vi "Get Loaded Instrument Configurations.vi"(8 "Error In":errorcluster) -> (0 "Error Out":errorcluster, 1 "Instrument Configurations":refnum<class "Config from JSON.lvclass">[](array[class]), 2 "Identifiers":string[](array[string]))   [LabVIEW 2020, in "Instrument Manager.lvclass"]
uses:
  Instrument Manager.lvclass
  Instrument Manager.lvclass/Instrument Manager.ctl
  Config from JSON/Config from JSON.lvclass
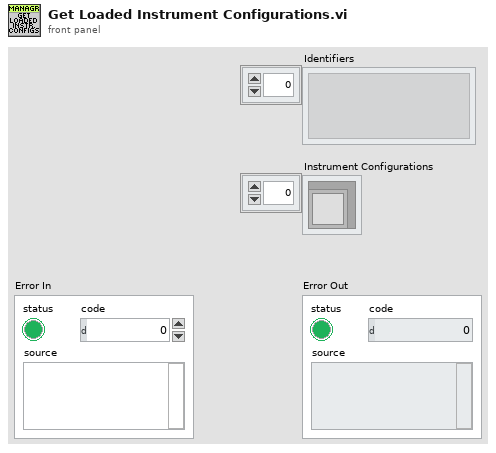
[diagram p1: front panel]
types:
  T1 = typedef "Instrument Manager.lvclass/ObjectAttributes.ctl" = cluster{"ICreate Action Point":refnum<class "ICreate Action Point.lvclass">, "IInstruments":map{string, refnum<class "IInstrument.lvclass">}, "IVirtual Instruments":map{string, refnum<class "IVirtual Instrument.lvclass">}, "Instrument Configurations":map{string, refnum<class "Config from JSON.lvclass">}, "Virtual Instrument Configurations":map{string, refnum<class "Config from JSON.lvclass">}, "Action Point Configurations":map{string, refnum<class "Config from JSON.lvclass">}, "Action Points":map{string, refnum<class "Action Point.lvclass">}}
  T2 = map{string, refnum<class "Config from JSON.lvclass">}
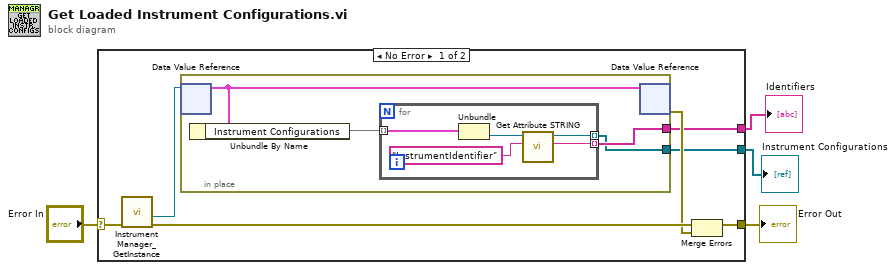
[diagram p0: block diagram]
diagram:
  n1 = case shown="No Error" "Error In" {
    selector: "Error In" -> [w11 w21]
    tunnel: [w9 w21] -> w3
    tunnel: [w6 _] -> w2
    tunnel: [w5 _] -> w1
    frame No Error {
      n2 = call "Instrument Manager_GetInstance.vi"("Error In"=w11) -> ("Error Out"=w10:errorcluster, "DVRRefOut"=w7:refnum<data-value>)  [unwired: 6 in, 3 out]
      n3 = in-place {
        in-place-border: [w14] -> w6
        in-place-border: [w13] -> w5
        n4 = in-place-dvr #1(w7) -> (w12:T1)  [unwired: 1 out]
        n5 = Unbundle By Name(w12) -> ("Instrument Configurations"=w15:T2)
        n6 = for {
          tunnel: w15 -> [w20] mode=indexing
          tunnel: [w17] -> w14 mode=indexing
          tunnel: [w16] -> w13 mode=indexing
          n7 = Unbundle(w20) -> ("Config from JSON.lvclass"=w19:refnum<class "Config from JSON.lvclass">)  [unwired: 1 out]
          n8 = call-dynamic "Get Attribute STRING.vi"("Attribute"="InstrumentIdentifier", "ConfigFromJSON in"=w19) -> ("Value"=w17:string, "ConfigFromJSON out"=w16:refnum<class "Config from JSON.lvclass">)  [unwired: 7 in, 1 out]
        }
        n9 = in-place-dvr #1(w12) -> (w8:errorcluster)  [unwired: 1 out]
      }
      n10 = Merge Errors(w10, w8) -> (w9:errorcluster)
    }
    frame Error {
    }
  }
  "Error Out" <- w3
  "Identifiers" <- w2
  "Instrument Configurations" <- w1
